vi "StartUp Sequence Open Loop Rev 1.7.vi"() -> ()   [LabVIEW 2017]
uses:
  <vilib>/addons/control/pid/pid.llb/PID (DBL).vi
  <vilib>/addons/control/pid/NI_PID_pid.lvlib
panel:
  out "Process variable and Setpoint":cluster{dbl, "Requested RPM (thousands):":dbl}(graph)
  in  "PID gains":T1={"proportional gain (Kc)"=0.6, "integral time (Ti, min)"=0.2, "derivative time (Td, min)"=0.0} {"derivative time (Td, min)" format="%.3f"; "integral time (Ti, min)" format="%.3f"; "proportional gain (Kc)" format="%.3f"}
  out "Measured RPM (thousands):":dbl(slide)=60.754431603254424 scale=44.0..130.0
  in  "Requested RPM (thousands):":dbl(slide)=45.0 min=0.0 max=0.0 scale=44.0..130.0
  out "MV:":dbl(slide)=18.78965245852964 scale=80.0..150.0
  out "Manipulated variable":i32(graph)
  out "Pump Enable":string
  in  "Soft Shut Off":bool
  out "Pump PWM":string
  in  "Send Command":bool
  in  "Custom Command":string
  out "Startup Success":bool
  in  "Output File":path
  in  "Emergency Shut Off":bool
  out "ECU COM Port Out":refnum<visa-resource-name>
  out "Turbine RPM":string
  out "Turbine Temp":string
  out "Error Out":errorcluster
  in  "Error In":errorcluster
  in  "ECU COM Port":refnum<visa-resource-name>
  out "Turbine State":string
  in  "Start Sequence":bool
  # "Note: save to a .csv file"
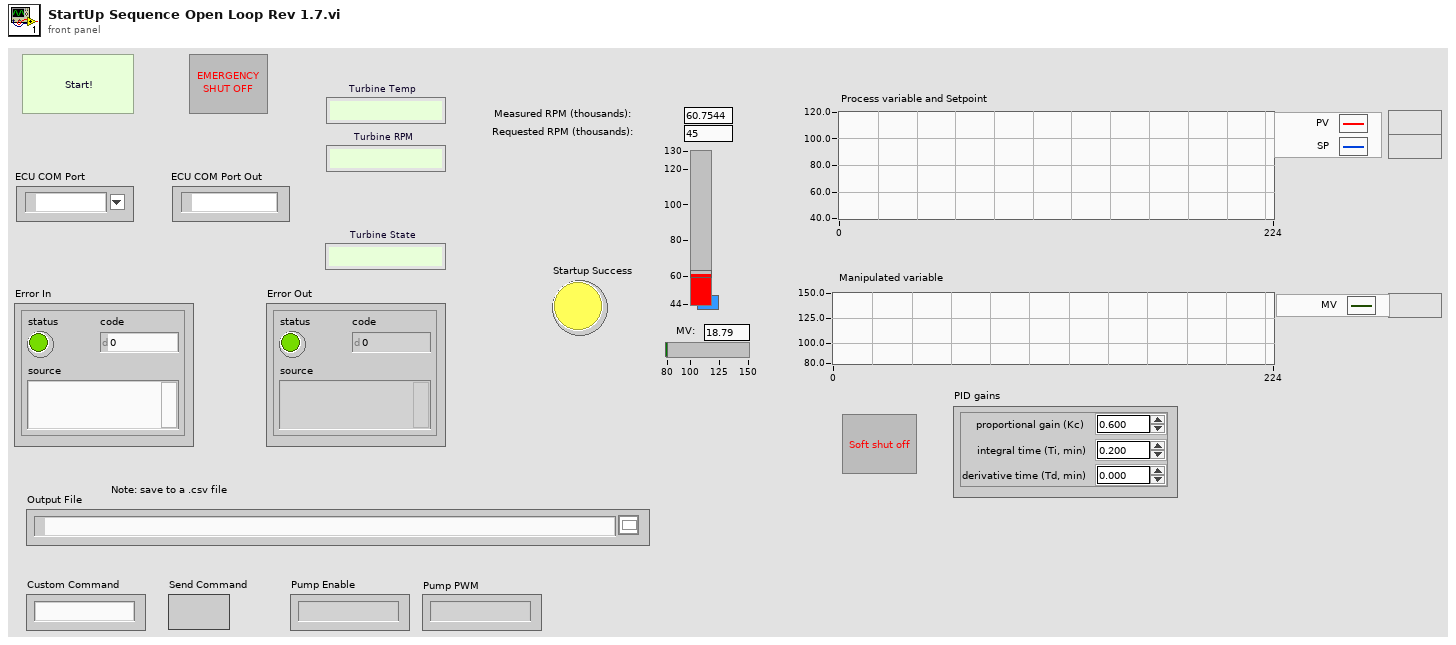
[diagram p1: front panel]
types:
  T1 = cluster{"proportional gain (Kc)":dbl, "integral time (Ti, min)":dbl, "derivative time (Td, min)":dbl}
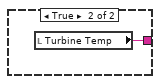
[diagram p3: hidden frame]
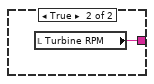
[diagram p4: hidden frame]
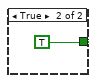
[diagram p7: hidden frame]
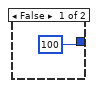
[diagram p8: hidden frame]
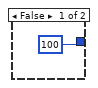
[diagram p9: hidden frame]
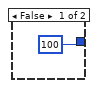
[diagram p10: hidden frame]
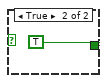
[diagram p11: hidden frame]
diagram:
  w30 = 21 ("Pulse Width")
  w31 = 160 ("Voltage")
  w35 = 16 ("Pulse Width")
  w36 = 160 ("Voltage")
  w27 = 255 ("y")
  w28 = 80 ("y")
  # "Increase fuel\nflow rate"
  # "Waits for the engine to reach\n44000 RPM"
  # "Ramp up the fuel flow rate\naccording to the current RPM.\nWaits until the RPMs reaches 40000"
  # "Ramp up the fuel valve to 66%\nand ramp up the fuel flow rate"
  # "Ramp up the fuel valve to 36%\nand the burner valve to 100%"
  # "Wait for temperature to reach 90 C"
  # "Ramp up the burner valve \nto 59%"
  # "Wait for temperature to reach 25 C"
  # "Update the pump values"
  # "Waits for the turbine to reach 3300 RPM"
  # "If the emergency shutoff button is pressed,\nthe engine will get shut down and the VI\nwill stop"
  # "Reset the Start Sequence\nbutton to false"
  # "Disengage Starter Motor"
  # "Starter Motor 55%"
  # "Start button is inside a while loop that doesn't progess until True"
  # "Fuel Pump Mode 2"
  # "GlowPlugOff"
  # "Start Up\nFuel Pump"
  n1 = call "Initialize Com Port.vi"("Error In"="Error In", "ECU COM Port"="ECU COM Port") -> ("Error Out"=w46:errorcluster, "ECU COM Port Out"=w45:refnum<visa-resource-name>)  [unwired: 8 in]
  n2 = while {
    tunnel: w46 -> [w99]
    tunnel: [w99] -> w44
    stop <- "Start Sequence" stop-if-true
  }
  n3 = call "Initialize Output File.vi"("error in (no error)"=w44, "Output File"="Output File") -> ("error out"=w26:errorcluster)  [unwired: 9 in]
  n4 = flat-sequence {
    tunnel: [w102] -> w25
    tunnel: w26 -> [w102]
    frame #0 {
      w101 = "0" ("Pump Value 1")
      n5 = local write "Pump Enable"(w101) -> ()
      n6 = local write "Pump PWM"(w101) -> ()
    }
  }
  n7 = flat-sequence {
    tunnel: w26 -> [w103]
    tunnel: [w103] -> w40
    frame #0 {
      n8 = local write "Start Sequence"(FALSE ("Strt Sqnc")) -> ()
    }
  }
  n9 = while {
    tunnel: ["Emergency Shut Off"] -> w96
    tunnel: "ECU COM Port" -> [w105]
    stop <- "Emergency Shut Off" stop-if-true
    n10 = case shown="True" "Emergency Shut Off" {
      tunnel: w105 -> [_ w109]
      frame False {
      }
      frame True {
        n11 = call "Emergency Shutoff.vi"("ECU COM Port"=w109) -> ("Error Out"=w108:errorcluster)  [unwired: 9 in, 1 out]
        n12 = local write "Output File"(path "" ("Output File")) -> ()
        n13 = flat-sequence {
          tunnel: w108 -> [w110]
          tunnel: [w110] -> _
          frame #0 {
            n14 = local write "Start Sequence"(FALSE ("Strt Sqnc")) -> ()
          }
        }
      }
    }
  }
  n15 = while {
    tunnel: w25 -> [w129]
    tunnel: w45 -> [w128]
    tunnel: "Output File" -> [w125]
    stop <- w124 continue-if-true
    n16 = call "Get Engine Update.vi"("Error In"=w129, "ECU COM Port"=w128) -> ("Error Out"=w126:errorcluster, "Temperature"=w118:string, "RPMs"=w112:string, "ECU COM Port Out"=w123:refnum<visa-resource-name>)  [unwired: 6 in]
    n17 = call "Time Delay4"() -> ()  [unwired: 11 in, 1 out]
    n18 = call "Safety Check.vi"("Temperature"=w118, "RPMs"=w112) -> ("Safe?"=w124:bool)  [unwired: 9 in]
    n19 = call "Error Check.vi"("Input"=w112) -> ("Error"=w113:bool)  [unwired: 10 in]
    n20 = call "Error Check.vi"("Input"=w118) -> ("Error"=w117:bool)  [unwired: 10 in]
    n21 = case shown="False" w124 {
      selector: w124 -> [w134 w136]
      tunnel: w123 -> [w135 _]
      tunnel: [w134 w136] -> w122
      frame False {
        n22 = call "Emergency Shutoff.vi"("ECU COM Port"=w135) -> ()  [unwired: 9 in, 2 out]
      }
      frame True {
      }
    }
    n23 = case shown="False" w113 {
      tunnel: w112 -> [w132 _]
      tunnel: [w132 w133] -> w115
      frame False {
        "Turbine RPM" <- w132
      }
      frame True {
        n24 = local read "Turbine RPM"() -> (w133:string)
      }
    }
    n25 = case shown="False" w117 {
      tunnel: w118 -> [w130 _]
      tunnel: [w130 w131] -> w119
      frame False {
        "Turbine Temp" <- w130
      }
      frame True {
        n26 = local read "Turbine Temp"() -> (w131:string)
      }
    }
    n27 = Not(x=w122) -> (.not. x?=w127:bool)
    n28 = local read "Requested RPM (thousands):"() -> (w116:dbl)
    n29 = Stop(stop? (T)=w127) -> ()
    n30 = local read "Pump Enable"() -> (w120:string)
    n31 = local read "Pump PWM"() -> (w121:string)
    n32 = Number To Decimal String(number=w116) -> (decimal integer string=w114:string)  [unwired: 1 in]
    n33 = call "Write Data to Output File.vi"("Pump Enable"=w120, "Requested RPM"=w114, "Pump PWM"=w121, "Error In"=w126, "Temperature"=w119, "RPM"=w115, "File Path Control"=w125) -> ()  [unwired: 4 in, 1 out]
  }
  n34 = call "Set Glow Plug Duty Cycle.vi"("Error In"=w40, "Duty Cycle"=6, "ECU COM Port"=w45) -> ("Error Out"=w88:errorcluster, "ECU COM Port Out"=w85:refnum<visa-resource-name>)  [unwired: 7 in]
  n35 = flat-sequence {
    tunnel: w40 -> [_]
    frame #0 {
      n36 = local write "Turbine State"("Initializing Motor") -> ()
    }
  }
  n37 = while {
    tunnel: w45 -> [w139]
    tunnel: w46 -> [_]
    stop <- FALSE stop-if-true
    n38 = case shown="True" "Send Command" {
      tunnel: "Custom Command" -> [_ w143]
      tunnel: w139 -> [_ w142]
      frame False {
      }
      frame True {
        n39 = call "Time Delay3"() -> ()  [unwired: 11 in, 1 out]
        n40 = VISA Write(VISA resource name=w142, write buffer=w143) -> ()  [unwired: 1 in, 3 out]
      }
    }
  }
  n41 = call "Delay"("error in (no error)"=w88, "Delay Time (s)"=2.0) -> ("error out"=w87:errorcluster)  [unwired: 9 in]
  n42 = call "Set Glow Plug Duty Cycle.vi"("Error In"=w87, "Duty Cycle"=19, "ECU COM Port"=w85) -> ("Error Out"=w86:errorcluster, "ECU COM Port Out"=w81:refnum<visa-resource-name>)  [unwired: 7 in]
  n43 = call "Delay"("error in (no error)"=w86, "Delay Time (s)"=3.0) -> ("error out"=w82:errorcluster)  [unwired: 9 in]
  n44 = call "Set Starter Motor Duty Cycle.vi"("Error In"=w82, "Duty Cycle"=6, "ECU COM Port"=w81) -> ("Error Out"=w80:errorcluster, "ECU COM Port Out"=w78:refnum<visa-resource-name>)  [unwired: 7 in]
  n45 = Stop(stop? (T)=w96) -> ()
  n46 = call "Set Glow Plug Duty Cycle.vi"("Error In"=w80, "Duty Cycle"=15, "ECU COM Port"=w78) -> ("Error Out"=w79:errorcluster, "ECU COM Port Out"=w74:refnum<visa-resource-name>)  [unwired: 7 in]
  n47 = call "Delay"("error in (no error)"=w79, "Delay Time (s)"=3.0) -> ("error out"=w76:errorcluster)  [unwired: 9 in]
  n48 = call "Set Starter Motor Duty Cycle.vi"("Error In"=w76, "Duty Cycle"=4, "ECU COM Port"=w74) -> ("Error Out"=w75:errorcluster, "ECU COM Port Out"=w73:refnum<visa-resource-name>)  [unwired: 7 in]
  n49 = call "Delay"("error in (no error)"=w75, "Delay Time (s)"=0.5) -> ("error out"=w97:errorcluster)  [unwired: 9 in]
  n50 = flat-sequence {
    tunnel: w97 -> [_]
    frame #0 {
      n51 = local write "Turbine State"("Check RPM") -> ()
    }
  }
  n52 = while {
    tunnel: w97 -> [w147]
    tunnel: w73 -> [w146]
    tunnel: [w146] -> w38
    tunnel: [w147] -> w98
    stop <- w150 stop-if-true
    n53 = local read "Turbine RPM"() -> (w145:string)
    n54 = Decimal String To Number(string=w145) -> (number=w149:i32)  [unwired: 2 in, 1 out]
    n55 = Greater Or Equal?(x=w149, y=3300) -> (x >= y?=w151:bool)
    n56 = case shown="False" w151 {
      tunnel: [FALSE TRUE] -> w150
      frame False {
        n57 = call "Delay2"() -> ()  [unwired: 11 in, 1 out]
      }
      frame True {
      }
    }
  }
  n58 = call "Set Pump Fow Rate.vi"("Error In"=w98, "Enable"=w35, "PWM"=w36, "ECU COM Port"=w38) -> ("Error Out"=w39:errorcluster, "ECU COM Port Out"=w37:refnum<visa-resource-name>)  [unwired: 6 in]
  n59 = flat-sequence {
    tunnel: w36 -> [w155]
    tunnel: w35 -> [w154]
    tunnel: w98 -> [_]
    frame #0 {
      n60 = Number To Decimal String(number=w154) -> (decimal integer string=w156:string)  [unwired: 1 in]
      n61 = Number To Decimal String(number=w155) -> (decimal integer string=w157:string)  [unwired: 1 in]
      n62 = local write "Pump Enable"(w156) -> ()
      n63 = local write "Pump PWM"(w157) -> ()
    }
  }
  n64 = call "Set Burner Valve Percent.vi"("Error In"=w39, "Percent"=10, "ECU COM Port"=w37) -> ("Error Out"=w10:errorcluster, "ECU COM Port Out"=w11:refnum<visa-resource-name>)  [unwired: 7 in]
  n65 = while {
    tunnel: [w159] -> w9
    tunnel: w10 -> [w159]
    tunnel: [w158] -> w8
    tunnel: w11 -> [w158]
    stop <- w160 stop-if-true
    n66 = local read "Turbine Temp"() -> (w163:string)
    n67 = Decimal String To Number(string=w163) -> (number=w162:i32)  [unwired: 2 in, 1 out]
    n68 = Greater?(x=w162, y=25) -> (0:w160:bool)
  }
  n69 = for {
    N: 8 -> [_]
    shift-right: [w169] -> _
    shift-left: 27 ("Percent") -> [w171]
    tunnel: w8 -> [w168]
    tunnel: w9 -> [w167]
    tunnel: [w164] -> w17
    tunnel: [w166] -> w18
    n70 = Add(x=w171, y=4 ("Percent")) -> (x+y=w169:i32)
    n71 = call "CmdSeparator"("Delay Time (s)"=0.5) -> ()  [unwired: 10 in, 1 out]
    n72 = call "Set Burner Valve Percent.vi"("Error In"=w167, "Percent"=w169, "ECU COM Port"=w168) -> ("Error Out"=w164:errorcluster, "ECU COM Port Out"=w166:refnum<visa-resource-name>)  [unwired: 7 in]
  }
  n73 = while {
    tunnel: w18 -> [w173]
    tunnel: w17 -> [w174]
    tunnel: [w173] -> w67
    tunnel: [w174] -> w68
    stop <- w177 stop-if-true
    # "Stage2Temp(C)"
    n74 = local read "Turbine Temp"() -> (w172:string)
    n75 = Decimal String To Number(string=w172) -> (number=w175:i32)  [unwired: 2 in, 1 out]
    n76 = Greater Or Equal?(x=w175, y=90) -> (x >= y?=w178:bool)
    n77 = case shown="False" w178 {
      tunnel: [FALSE TRUE] -> w177
      frame False {
        n78 = call "Delay3"() -> ()  [unwired: 11 in, 1 out]
      }
      frame True {
      }
    }
  }
  n79 = flat-sequence {
    tunnel: w17 -> [_]
    frame #0 {
      n80 = local write "Turbine State"("Check Temp") -> ()
    }
  }
  n81 = call "Set Glow Plug Duty Cycle.vi"("Error In"=w68, "Duty Cycle"=0, "ECU COM Port"=w67) -> ("Error Out"=w66:errorcluster, "ECU COM Port Out"=w32:refnum<visa-resource-name>)  [unwired: 7 in]
  n82 = call "CmdSeparator3"("error in (no error)"=w66, "Delay Time (s)"=0.2) -> ("error out"=w29:errorcluster)  [unwired: 9 in]
  n83 = call "Set Pump Fow Rate.vi"("Error In"=w29, "Enable"=w30, "PWM"=w31, "ECU COM Port"=w32) -> ("Error Out"=w34:errorcluster, "ECU COM Port Out"=w33:refnum<visa-resource-name>)  [unwired: 6 in]
  n84 = call "Set Burner Valve Percent.vi"("Error In"=w34, "Percent"=80, "ECU COM Port"=w33) -> ("Error Out"=w63:errorcluster, "ECU COM Port Out"=w64:refnum<visa-resource-name>)  [unwired: 7 in]
  n85 = flat-sequence {
    tunnel: w31 -> [w183]
    tunnel: w30 -> [w182]
    tunnel: w29 -> [_]
    frame #0 {
      n86 = Number To Decimal String(number=w182) -> (decimal integer string=w184:string)  [unwired: 1 in]
      n87 = Number To Decimal String(number=w183) -> (decimal integer string=w185:string)  [unwired: 1 in]
      n88 = local write "Pump Enable"(w184) -> ()
      n89 = local write "Pump PWM"(w185) -> ()
    }
  }
  n90 = call "CmdSeparator18"("error in (no error)"=w63, "Delay Time (s)"=0.75) -> ("error out"=w62:errorcluster)  [unwired: 9 in]
  n91 = call "Set Fuel Valve Percent.vi"("Error In"=w62, "Percent"=12, "ECU COM Port"=w64) -> ("Error Out"=w61:errorcluster, "ECU COM Port Out"=w65:refnum<visa-resource-name>)  [unwired: 7 in]
  n92 = call "CmdSeparator16"("error in (no error)"=w61, "Delay Time (s)"=0.2) -> ("error out"=w94:errorcluster)  [unwired: 9 in]
  n93 = for {
    N: 4 -> [_]
    tunnel: [w187] -> _
    tunnel: [w201] -> _
    tunnel: w65 -> [w193]
    tunnel: w94 -> [w194]
    shift-right: [w192] -> w57
    shift-left: 12 -> [w198]
    shift-right: [w189] -> _
    shift-left: 80 -> [w195]
    tunnel: [w201] -> w55 mode=indexing
    tunnel: [w187] -> w58 mode=indexing
    n94 = Less?(x=w198, y=100) -> (x < y?=w199:bool)
    n95 = Less?(x=w195, y=100) -> (x < y?=w196:bool)
    n96 = case shown="True" w196 {
      tunnel: w195 -> [_ w205]
      tunnel: [100 w203] -> w189
      frame False {
      }
      frame True {
        n97 = Add(x=w205, y=5) -> (x+y=w203:i32)
      }
    }
    n98 = case shown="True" w199 {
      tunnel: w198 -> [_ w209]
      tunnel: [100 w207] -> w192
      frame False {
      }
      frame True {
        n99 = Add(x=w209, y=6) -> (x+y=w207:i32)
      }
    }
    n100 = call "Set Fuel Valve Percent.vi"("Error In"=w194, "Percent"=w192, "ECU COM Port"=w193) -> ("Error Out"=w191:errorcluster, "ECU COM Port Out"=w188:refnum<visa-resource-name>)  [unwired: 7 in]
    n101 = call "Set Burner Valve Percent.vi"("Error In"=w191, "Percent"=w189, "ECU COM Port"=w188) -> ("Error Out"=w190:errorcluster, "ECU COM Port Out"=w187:refnum<visa-resource-name>)  [unwired: 7 in]
    n102 = call "CmdSeparator17"("error in (no error)"=w190, "Delay Time (s)"=0.75) -> ("error out"=w201:errorcluster)  [unwired: 9 in]
  }
  n103 = flat-sequence {
    tunnel: w55 -> [_]
    frame #0 {
      n104 = local write "Turbine State"("Pump Ramp Up") -> ()
    }
  }
  n105 = for {
    N: 3 -> [_]
    tunnel: [w218] -> w48
    tunnel: [w229] -> w49
    shift-right: [w225] -> _
    shift-left: w57 -> [w226]
    tunnel: w55 -> [w222] mode=indexing
    tunnel: w58 -> [w221] mode=indexing
    shift-right: [w214] -> _
    shift-left: 21 -> [w215]
    w213 = 160 ("y")
    n106 = Less?(x=w226, y=100) -> (x < y?=w227:bool)
    n107 = Add(x=w215, y=1) -> (x+y=w214:i32)
    n108 = case shown="True" w227 {
      tunnel: w226 -> [_ w237]
      tunnel: [100 w235] -> w225
      frame False {
      }
      frame True {
        n109 = Add(x=w237, y=10) -> (x+y=w235:i32)
      }
    }
    n110 = call "Set Fuel Valve Percent.vi"("Error In"=w222, "Percent"=w225, "ECU COM Port"=w221) -> ("Error Out"=w224:errorcluster, "ECU COM Port Out"=w223:refnum<visa-resource-name>)  [unwired: 7 in]
    n111 = call "Set Burner Valve Percent.vi"("Error In"=w224, "Percent"=100 ("y"), "ECU COM Port"=w223) -> ("Error Out"=w212:errorcluster, "ECU COM Port Out"=w219:refnum<visa-resource-name>)  [unwired: 7 in]
    n112 = call "Set Pump Fow Rate.vi"("Error In"=w212, "Enable"=w214, "PWM"=w213, "ECU COM Port"=w219) -> ("Error Out"=w217:errorcluster, "ECU COM Port Out"=w218:refnum<visa-resource-name>)  [unwired: 6 in]
    n113 = flat-sequence {
      tunnel: w213 -> [w231]
      tunnel: w214 -> [w230]
      tunnel: w212 -> [_]
      frame #0 {
        n114 = Number To Decimal String(number=w230) -> (decimal integer string=w232:string)  [unwired: 1 in]
        n115 = Number To Decimal String(number=w231) -> (decimal integer string=w233:string)  [unwired: 1 in]
        n116 = local write "Pump Enable"(w232) -> ()
        n117 = local write "Pump PWM"(w233) -> ()
      }
    }
    n118 = call "CmdSeparator20"("error in (no error)"=w217, "Delay Time (s)"=0.5) -> ("error out"=w229:errorcluster)  [unwired: 9 in]
  }
  n119 = call "Set Starter Motor Duty Cycle.vi"("Error In"=w49, "Duty Cycle"=11, "ECU COM Port"=w48) -> ("Error Out"=w14:errorcluster, "ECU COM Port Out"=w15:refnum<visa-resource-name>)  [unwired: 7 in]
  n120 = while {
    tunnel: w15 -> [w243]
    tunnel: w14 -> [w242]
    tunnel: [w241] -> w12
    tunnel: [w240] -> w13
    stop <- w246 stop-if-true
    w245 = 160 ("y")
    n121 = local read "Turbine RPM"() -> (w252:string)
    n122 = Decimal String To Number(string=w252) -> (number=w248:i32)  [unwired: 2 in, 1 out]
    n123 = Multiply(x=w248, y=0.0008) -> (x*y=w250:dbl)
    n124 = call "Set Fuel Valve Percent.vi"("Error In"=w242, "Percent"=100 ("y"), "ECU COM Port"=w243) -> ("Error Out"=w257:errorcluster, "ECU COM Port Out"=w256:refnum<visa-resource-name>)  [unwired: 7 in]
    n125 = Add(x=w250, y=10.537) -> (x+y=w244:dbl)
    n126 = call "Set Burner Valve Percent.vi"("Error In"=w257, "Percent"=0 ("y"), "ECU COM Port"=w256) -> ("Error Out"=w253:errorcluster, "ECU COM Port Out"=w254:refnum<visa-resource-name>)  [unwired: 7 in]
    n127 = call "Set Pump Fow Rate.vi"("Error In"=w253, "Enable"=w244, "PWM"=w245, "ECU COM Port"=w254) -> ("Error Out"=w239:errorcluster, "ECU COM Port Out"=w241:refnum<visa-resource-name>)  [unwired: 6 in]
    n128 = call "CmdSeparator5"("error in (no error)"=w239, "Delay Time (s)"=0.25) -> ("error out"=w240:errorcluster)  [unwired: 9 in]
    n129 = flat-sequence {
      tunnel: w245 -> [w261]
      tunnel: w244 -> [w260]
      tunnel: [w259] -> _
      tunnel: w239 -> [w259]
      frame #0 {
        n130 = Number To Decimal String(number=w260) -> (decimal integer string=w262:string)  [unwired: 1 in]
        n131 = Number To Decimal String(number=w261) -> (decimal integer string=w263:string)  [unwired: 1 in]
        n132 = local write "Pump Enable"(w262) -> ()
        n133 = local write "Pump PWM"(w263) -> ()
      }
    }
    n134 = Greater Or Equal?(x=w248, y=40000) -> (x >= y?=w246:bool)
  }
  n135 = flat-sequence {
    tunnel: w14 -> [_]
    frame #0 {
      n136 = local write "Turbine State"("Ramp Up to Idle") -> ()
    }
  }
  n137 = call "Set Pump Fow Rate.vi"("Error In"=w13, "Enable"=w27, "PWM"=w28, "ECU COM Port"=w12) -> ("Error Out"=w16:errorcluster, "ECU COM Port Out"=w54:refnum<visa-resource-name>)  [unwired: 6 in]
  n138 = flat-sequence {
    tunnel: w28 -> [w267]
    tunnel: w27 -> [w266]
    tunnel: w16 -> [w265]
    tunnel: [w265] -> _
    frame #0 {
      n139 = Number To Decimal String(number=w266) -> (decimal integer string=w268:string)  [unwired: 1 in]
      n140 = Number To Decimal String(number=w267) -> (decimal integer string=w269:string)  [unwired: 1 in]
      n141 = local write "Pump Enable"(w268) -> ()
      n142 = local write "Pump PWM"(w269) -> ()
    }
  }
  n143 = while {
    tunnel: w16 -> [w271]
    tunnel: w54 -> [w270]
    tunnel: [w271] -> w51
    tunnel: [w270] -> w53
    stop <- w272 stop-if-true
    n144 = local read "Turbine RPM"() -> (w275:string)
    n145 = Decimal String To Number(string=w275) -> (number=w274:i32)  [unwired: 2 in, 1 out]
    n146 = Greater?(x=w274, y=44000) -> (0:w272:bool)
  }
  n147 = flat-sequence {
    tunnel: w51 -> [_]
    frame #0 {
      n148 = local write "Turbine State"("Normal Operation") -> ()
    }
  }
  n149 = call "Set Starter Motor Duty Cycle.vi"("Error In"=w51, "Duty Cycle"=0, "ECU COM Port"=w53) -> ("Error Out"=w23:errorcluster, "ECU COM Port Out"=w24:refnum<visa-resource-name>)  [unwired: 7 in]
  n150 = flat-sequence {
    tunnel: w23 -> [_]
    frame #0 {
      "Startup Success" <- TRUE
    }
  }
  n151 = while {
    tunnel: [w293] -> w22
    tunnel: [w292] -> w21
    tunnel: w24 -> [w290]
    tunnel: w23 -> [w291]
    stop <- "Soft Shut Off" stop-if-true
    # "Control loop using PID"
    n152 = local read "Turbine RPM"() -> (w289:string)
    n153 = Decimal String To Number(string=w289) -> (number=w286:i32)  [unwired: 2 in, 1 out]
    n154 = Divide(x=w286, y=1000) -> (x/y=w278:dbl)
    "Measured RPM (thousands):" <- w278
    n155 = Wait Until Next ms Multiple(millisecond multiple=u32 500 ("unsigned 32bit integer")) -> ()  [unwired: 1 out]
    n156 = call-poly <vilib>:"PID.vi"("output range"=cluster{"output high":dbl, "output low":dbl} {"output high"=20.0, "output low"=-20.0}, "PID gains"="PID gains", "process variable"=w278, "setpoint"="Requested RPM (thousands):") -> ("output"=w282:dbl)  [unwired: 6 in, 1 out]
    n157 = Add(x=w278, y=w282) -> (x+y=w281:dbl)
    n158 = Multiply(x=w281, y=1000.0) -> (x*y=w280:dbl)
    n159 = Bundle(w278, "Requested RPM (thousands):"="Requested RPM (thousands):") -> (→"Process variable and Setpoint":cluster{dbl, "Requested RPM (thousands):":dbl})  [unwired: 1 in]
    n160 = call "RPM to Fuel Flow.vi"("Requested RPM"=w280) -> ("Fuel Pump PWM"=w283:i32)  [unwired: 10 in]
    "MV:" <- w283
    "Manipulated variable" <- w283
    n161 = Number To Decimal String(number=w283) -> (decimal integer string=→"Pump PWM":string)  [unwired: 1 in]
    n162 = call "Set Pump Fow Rate.vi"("Error In"=w291, "Enable"=255 ("Pulse Width"), "PWM"=w283, "ECU COM Port"=w290) -> ("Error Out"=w292:errorcluster, "ECU COM Port Out"=w293:refnum<visa-resource-name>)  [unwired: 6 in]
    n163 = local write "Pump Enable"("255" ("Pump Value 2")) -> ()
  }
  n164 = call "Emergency Shutoff.vi"("Error In"=w21, "ECU COM Port"=w22) -> ("Error Out"=w42:errorcluster, "ECU COM Port Out"=→"ECU COM Port Out":refnum<visa-resource-name>)  [unwired: 8 in]
  n165 = flat-sequence {
    tunnel: w42 -> [w301]
    tunnel: [w301] -> w95
    frame #0 {
      w300 = "0"
      n166 = local write "Pump Enable"(w300) -> ()
      n167 = local write "Pump PWM"(w300) -> ()
    }
  }
  "Error Out" <- w95
